vi "TSM SSC DCPower Query Output State.vi"(0 "DCPower TSM in":T2, 5 "Output State":T1 items=["Constant Voltage", "Constant Current"], 11 "error in":errorcluster) -> (4 "DCPower TSM out":T2, 6 "In State?":bool[](array[boolean]), 15 "error out":errorcluster)   [LabVIEW 2020]
doc: "Queries the specified output channel to determine if the output channels are currently in the state specified by <B>output state</B>."
uses:
  TSM/TSM SSC DCPower.ctl
  <vilib>/NI_TestStand_SemiconductorModule/NI_TestStand_Semiconductor_Module.lvlibp/PinMap/PinQueryContext/MultiplePinMultipleSessionQueryContext/MultiplePinMultipleSessionQueryContext.lvclass
  SSC DCPower/SSC DCPower.ctl
  Shared SubVIs/TSM Pin Abstraction/TSM Pin Information.ctl
  Shared SubVIs/TSM Pin Abstraction/TSM Pin Type Identifier.ctl
  Shared SubVIs/TSM Pin Abstraction/TSM Expanded Pin Information.ctl
  <instrlib>/niDCPower/nidcpower.llb/niDCPower Output State.ctl
  <instrlib>/niDCPower/nidcpower.llb/niDCPower Query Output State.vi
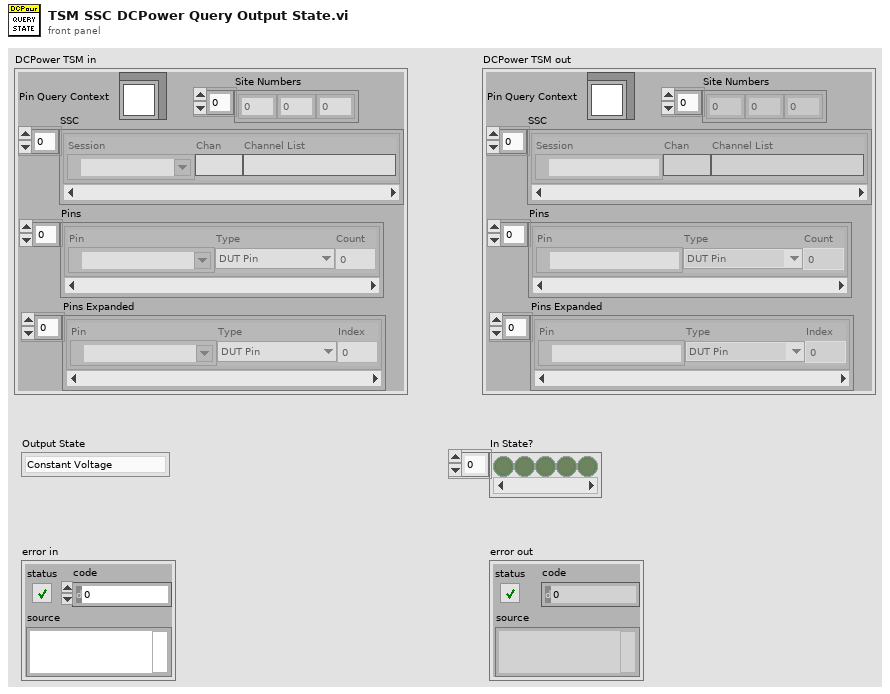
[diagram p1: front panel]
types:
  T1 = typedef "niDCPower Output State.ctl" = u16
  T2 = typedef "TSM SSC DCPower.ctl" = cluster{"Pin Query Context":refnum<class "MultiplePinMultipleSessionQueryContext.lvclass">, "SSC":T3[], "Site Numbers":i32[], "Pins":T4[], "Pins Expanded":T6[]}
  T3 = typedef "SSC DCPower.ctl" = cluster{"Session":refnum<k15>, "Chan":string, "Channel List":string}
  T4 = typedef "TSM Pin Information.ctl" = cluster{"Pin":tag, "Type":T5, "Count":i32}
  T5 = typedef "TSM Pin Type Identifier.ctl" = enum8{"DUT Pin", "System Pin", "Pin Group", "Not Determined"}
  T6 = typedef "TSM Expanded Pin Information.ctl" = cluster{"Pin":tag, "Type":T5, "Index":i32}
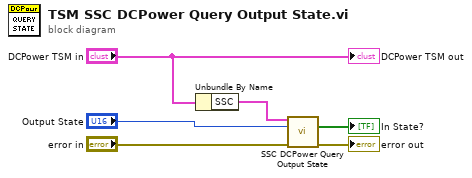
[diagram p0: block diagram]
diagram:
  n1 = Unbundle By Name("DCPower TSM in") -> ("SSC"=w3:T3[])
  n2 = call "SSC DCPower Query Output State.vi"("DCPower SSC in"=w3, "Output State"="Output State", "error in"="error in") -> ("In State?"=→"In State?":bool[], "error out"=→"error out":errorcluster)  [unwired: 10 in, 1 out]
  "DCPower TSM out" <- "DCPower TSM in"
